vi "filemove.vi"(8 "错误输入":errorcluster, 9 "清空":bool, 10 "目标路径":path, 11 "源路径":path) -> (0 "错误输出":errorcluster, 2 "msg":string, 3 "新路径":path)   [LabVIEW 2011]
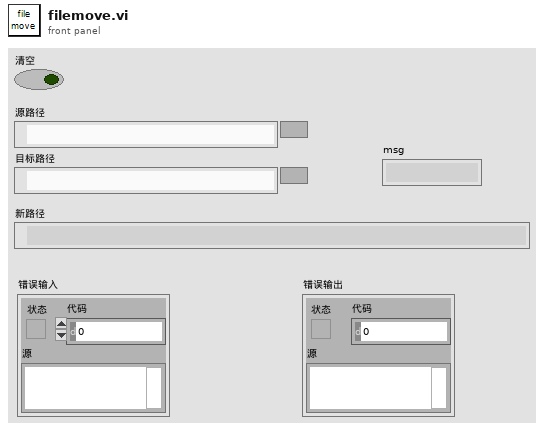
[diagram p1: front panel]
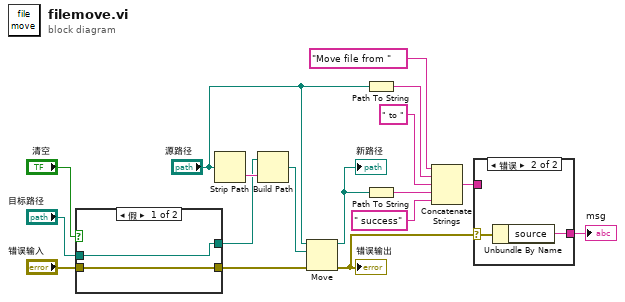
[diagram p0: block diagram]
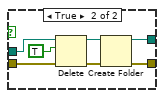
[diagram p2: hidden frame]
diagram:
  n1 = case shown="假" "清空" {
    tunnel: "目标路径" -> [w19 w23]
    tunnel: [w19 w22] -> w15
    tunnel: [w18 w21] -> w13
    tunnel: "错误输入" -> [w18 w20]
    frame False {
    }
    frame True {
      n2 = Delete(path (use dialog)=w23, entire hierarchy (F)=TRUE ("整个层次结构(F)"), error in=w20) -> (deleted path=w25:path, error out=w24:errorcluster)  [unwired: 2 in, 1 out]
      n3 = Create Folder(path (use dialog)=w25, error in=w24) -> (created path=w22:path, error out=w21:errorcluster)  [unwired: 1 in, 1 out]
    }
  }
  n4 = Strip Path(path="源路径") -> (name=w17:string)  [unwired: 1 out]
  n5 = Build Path(base path=w15, name or relative path=w17) -> (appended path=w14:path)
  n6 = Move(source path="源路径", error in=w13, 10:w14) -> (error out=w11:errorcluster, 3:w9:path)  [unwired: 2 in, 1 out]
  "新路径" <- w9
  "错误输出" <- w11
  n7 = Path To String(path="源路径") -> (string=w7:string)
  n8 = Path To String(path=w9) -> (string=w5:string)
  n9 = Concatenate Strings("Move file from " ("字符串"), w7, " to " ("字符串"), w5, " success" ("字符串")) -> (w3:string)
  n10 = case shown="错误" w11 {
    selector: w11 -> [_ w29]
    tunnel: w3 -> [w27 _]
    tunnel: [w27 w28] -> w2
    frame No Error {
    }
    frame Error {
      n11 = Unbundle By Name(w29) -> ("source"=w28:string)
    }
  }
  "msg" <- w2
